vi "RSZVB Define Balanced Port.vi"(6 "Physical Port 1 (1)":i32=1, 7 "Physical Port 2 (1)":i32=1, 8 "error in (no error)":errorcluster {"code" format="%.0x"}, 9 "Logical Port (1)":i32=1, 10 "Channel (1)":i32=1, 11 "VISA session":refnum<visa-resource-name>) -> (0 "error out":errorcluster {"code" format="%.0x"}, 3 "dup VISA session":refnum<visa-resource-name>)   [LabVIEW 2011]
doc: "This VI defines a balanced port numbered <Logicalog Port>, combining two physical ports <Physical Port 1> and <Physical Port 2>.\n\nRemote-control command(s):\nSOURce<Ch>:LPORt<log_port>"
uses:
  _utility/RSZVB Global Data.vi
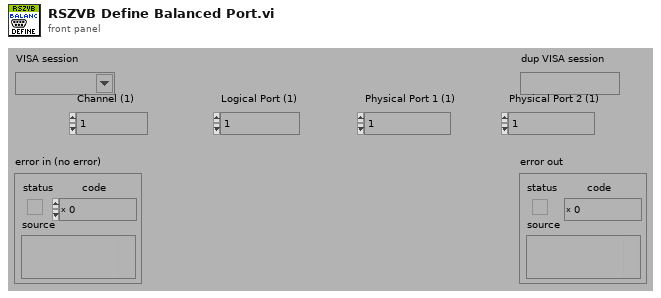
[diagram p1: front panel]
types:
  T1 = cluster{"Error Checking (T: On)":bool, "Installed Options":string[], "Data Valid?":bool, "Ports":i32, "Model":string[], "Option Checking (T: On)":bool}[]
  T2 = cluster{"Error Checking (T: On)":bool, "Installed Options":string[], "Data Valid?":bool, "Ports":i32, "Model":string[], "Option Checking (T: On)":bool}
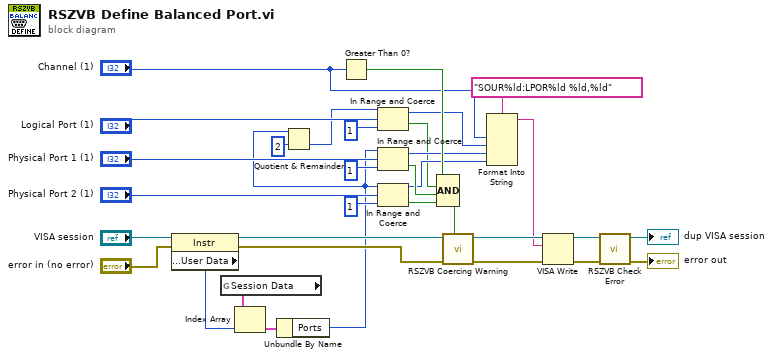
[diagram p0: block diagram]
diagram:
  n1 = property class="Instr"(reference="VISA session", error in="error in (no error)") -> (reference out=w19:refnum<visa-resource-name>, error out=w20:errorcluster, "General Settings:User Data"=w21:u32)
  n2 = global read "RSZVB Global Data.vi" "Session Data"() -> (w22:T1)
  n3 = Index Array(array=w22, index=w21) -> (element=w23:T2)
  n4 = Unbundle By Name(w23) -> ("Ports"=w2:i32)
  n5 = Quotient & Remainder(x=w2, y=2) -> (floor(x/y)=w3:i32)  [unwired: 1 out]
  n6 = Greater Than 0?(x="Channel (1)") -> (x > 0?=w24:bool)
  n7 = In Range and Coerce(upper limit=w3, x="Logical Port (1)", lower limit=1) -> (coerced(x)=w1:i32, In Range?=w6:bool)
  n8 = In Range and Coerce(upper limit=w2, x="Physical Port 1 (1)", lower limit=1) -> (coerced(x)=w16:i32, In Range?=w27:bool)
  n9 = In Range and Coerce(upper limit=w2, x="Physical Port 2 (1)", lower limit=1) -> (coerced(x)=w15:i32, In Range?=w17:bool)
  n10 = Compound Arithmetic op=AND(w24, w6, w27, w17) -> (w26:bool)
  n11 = call "RSZVB Coercing Warning.vi"("In Range?"=w26, "error in (no error)"=w20, "VISA session"=w19) -> ("error out"=w30:errorcluster, "dup VISA session"=w31:refnum<visa-resource-name>)  [unwired: 7 in]
  n12 = Format Into String(format string="SOUR%ld:LPOR%ld %ld,%ld", "Channel (1)", w1, w16, w15) -> (resulting string=w25:string)  [unwired: 2 in, 1 out]
  n13 = VISA Write(VISA resource name=w31, write buffer=w25, error in (no error)=w30) -> (VISA resource name out=w28:refnum<visa-resource-name>, error out=w29:errorcluster)  [unwired: 1 out]
  n14 = call "RSZVB Check Error.vi"("error in (no error)"=w29, "VISA session"=w28) -> ("error out"=→"error out":errorcluster, "dup VISA session"=→"dup VISA session":refnum<visa-resource-name>)  [unwired: 8 in]
